vi "CopyScriptFromPluginTreeToTestTree.vi"(8 "error in (no error)":errorcluster, 10 "PluginTree":refnum<vi>, 11 "TestListboxRef":refnum<vi>) -> (0 "error out":errorcluster, 1 "Added Script?":bool, 2 "All Tags":string[](array[string]))   [LabVIEW 2018]
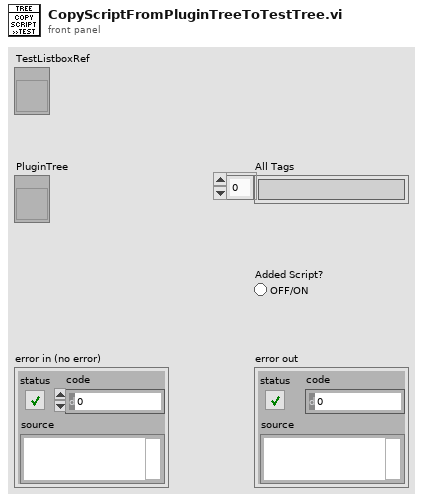
[diagram p1: front panel]
types:
  T1 = enum16{"Init Symbols", "Set Item Symbol", "Get Symbol Index"}
  T2 = typedef "Plugin Tree Tag.ctl" = cluster{"ItemType":T3, "Name":string, "Path":path, "Script":string[]}
  T3 = typedef "Plugins Tree Item Type.ctl" = enum16{"Plugin", "Instrument", "INI File", "INI Script"}
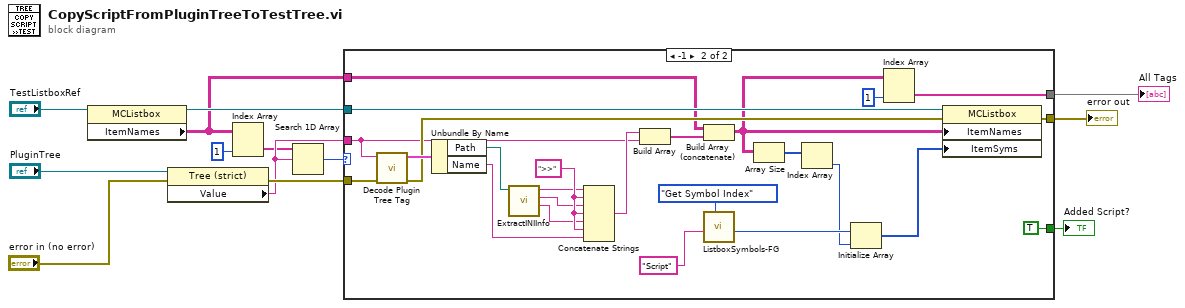
[diagram p0: block diagram]
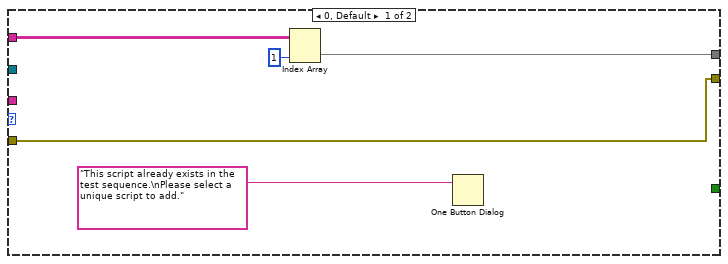
[diagram p2: hidden frame]
diagram:
  n1 = property class="MCListbox"(reference="TestListboxRef") -> (reference out=w9:refnum<vi>, "ItemNames"=w3:string[][])  [unwired: 1 in, 1 out]
  n2 = property class="Tree (strict)"(reference="PluginTree", error in="error in (no error)") -> (error out=w13:errorcluster, "Value"=w7:string)  [unwired: 1 out]
  n3 = Index Array(array=w3, index (col)=1 ("disabled index (col)")) -> (element=w4:string[])  [unwired: 1 in]
  n4 = Search 1D Array(1D array=w4, element=w7) -> (index of element=w8:i32)  [unwired: 1 in]
  n5 = case shown="-1" w8 {
    tunnel: w13 -> [w17 w41]
    tunnel: w7 -> [_ w31]
    tunnel: w9 -> [_ w34]
    tunnel: [_ TRUE] -> w6
    tunnel: w3 -> [w15 w21]
    tunnel: [w17 w23] -> w2
    tunnel: [w14 w20] -> w1
    frame 0, Default {
      n6 = Index Array(array=w15, index (col)=1 ("disabled index (col)")) -> (element=w14:string[])  [unwired: 1 in]
      n7 = One Button Dialog(message="This script already exists in the test sequence.\nPlease select a unique script to add.") -> ()  [unwired: 1 in, 1 out]
    }
    frame -1 {
      w43 = ">>" ("Module Name")
      n8 = call "Decode Plugin Tree Tag.vi"("error in (no error)"=w41, "Tag"=w31) -> ("error out"=w33:errorcluster, "Plugin Tree Tag"=w36:T2)  [unwired: 8 in]
      n9 = Unbundle By Name(w36) -> ("Path"=w37:path, "Name"=w42:string)
      n10 = call "ExtractINIInfo.vi"("INI File Path"=w37) -> ("INI File Name"=w40:string, "Instrument name"=w39:string, "Module Name"=w38:string)  [unwired: 5 in, 3 out]
      n11 = Concatenate Strings(w38, w43, w39, w43, w40, w43, w42) -> (w32:string)
      n12 = Build Array(w32, w31) -> (w28:string[])
      n13 = Build Array (concatenate)(w21, w28) -> (w19:string[][])
      n14 = call "ListboxSymbols-FG.vi"("Actions"=T1."Get Symbol Index", "Symbol Name"="Script") -> ("Symbol Index"=w26:i32)  [unwired: 6 in, 3 out]
      n15 = Array Size(array=w19) -> (size(s)=w27:i32[])
      n16 = Index Array(array=w27) -> (element=w25:i32)  [unwired: 1 in]
      n17 = Initialize Array(w26, w25) -> (w24:i32[])
      n18 = Index Array(array=w19, index (col)=1 ("disabled index (col)")) -> (element=w20:string[])  [unwired: 1 in]
      n19 = property class="MCListbox"(reference=w34, error in=w33, "ItemNames"=w19, "ItemSyms"=w24) -> (error out=w23:errorcluster)  [unwired: 1 out]
    }
  }
  "error out" <- w2
  "Added Script?" <- w6
  "All Tags" <- w1
